vi "Dpc Init.vi"(8 "error in (no error)":errorcluster, 11 "perc":i32) -> (0 "error out":errorcluster, 2 "function return":i32, 3 "perc out":i32)   [LabVIEW 2011, in "LVH-Adept.lvlib" / "DPCUTIL.lvlib"]
doc: "DPCAPI BOOL DpcInit(ERC * perc);"
uses:
  DPCUTIL.lvlib
  Resources/dpcutil.dll
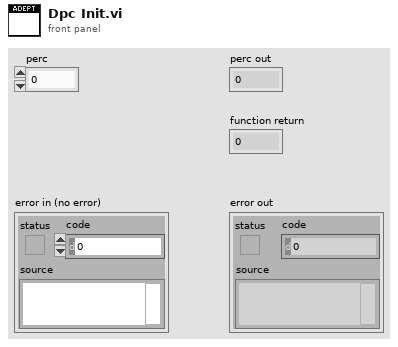
[diagram p1: front panel]
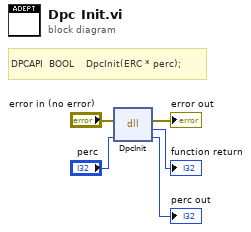
[diagram p0: block diagram]
diagram:
  # "DPCAPI  BOOL    DpcInit(ERC * perc);"
  n1 = dll-call lib="C:/github/labviewhacker/LVH-Adept/LabVIEW/vi.lib/LabVIEW Hacker/Adept/Private/Resources/dpcutil.*" fn="DpcInit"(error in="error in (no error)", "perc"="perc") -> (error out=→"error out":errorcluster, →"function return":i32, "perc"=→"perc out":i32)  [unwired: 2 in, 1 out]
